vi "Requests.vi"(8 "error in (no error)":errorcluster, 9 "write enable":bool=TRUE, 11 "TCP Client in":refnum<class "WebSocket Client CR.lvclass">) -> (0 "error out":errorcluster, 3 "MB_TCP out":refnum<class "WebSocket Client CR.lvclass">)   [LabVIEW 2021, in "WebSockets.lvlib" / "WebSocket Client CR.lvclass"]
uses:
  WebSocket Client CR.lvclass
  WebSocket/WebSocket.lvclass
  WebSocket Server/TCP Server/Handler State.ctl
  WebSocket Server/TCP Server/TCP Server.lvclass
  WebSocket/Opcodes.ctl
  Data Model/WebSocket Data Model.lvclass
  Modbus_v121c/Data Model/Device Data Model.lvclass
panel:
  out "Data":u8[](array[numeric])
  in  "stop":bool
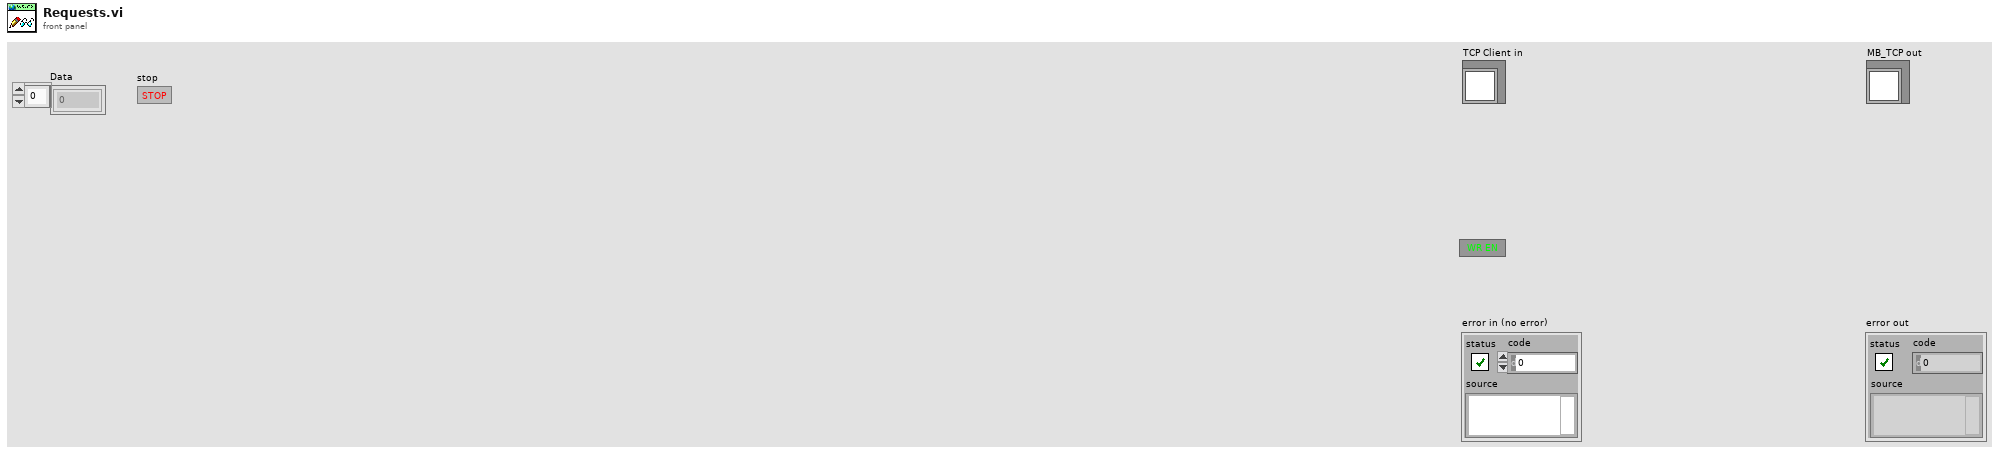
[diagram p1: front panel]
types:
  T1 = typedef "WebSockets.lvlib/WebSocket.lvclass/Opcodes.ctl" = u8
  T2 = typedef "WebSockets.lvlib/TCP Server.lvclass/Handler State.ctl" = enum16{"Wait on Connection", "Execute function", "Close Connection", "Quit"}
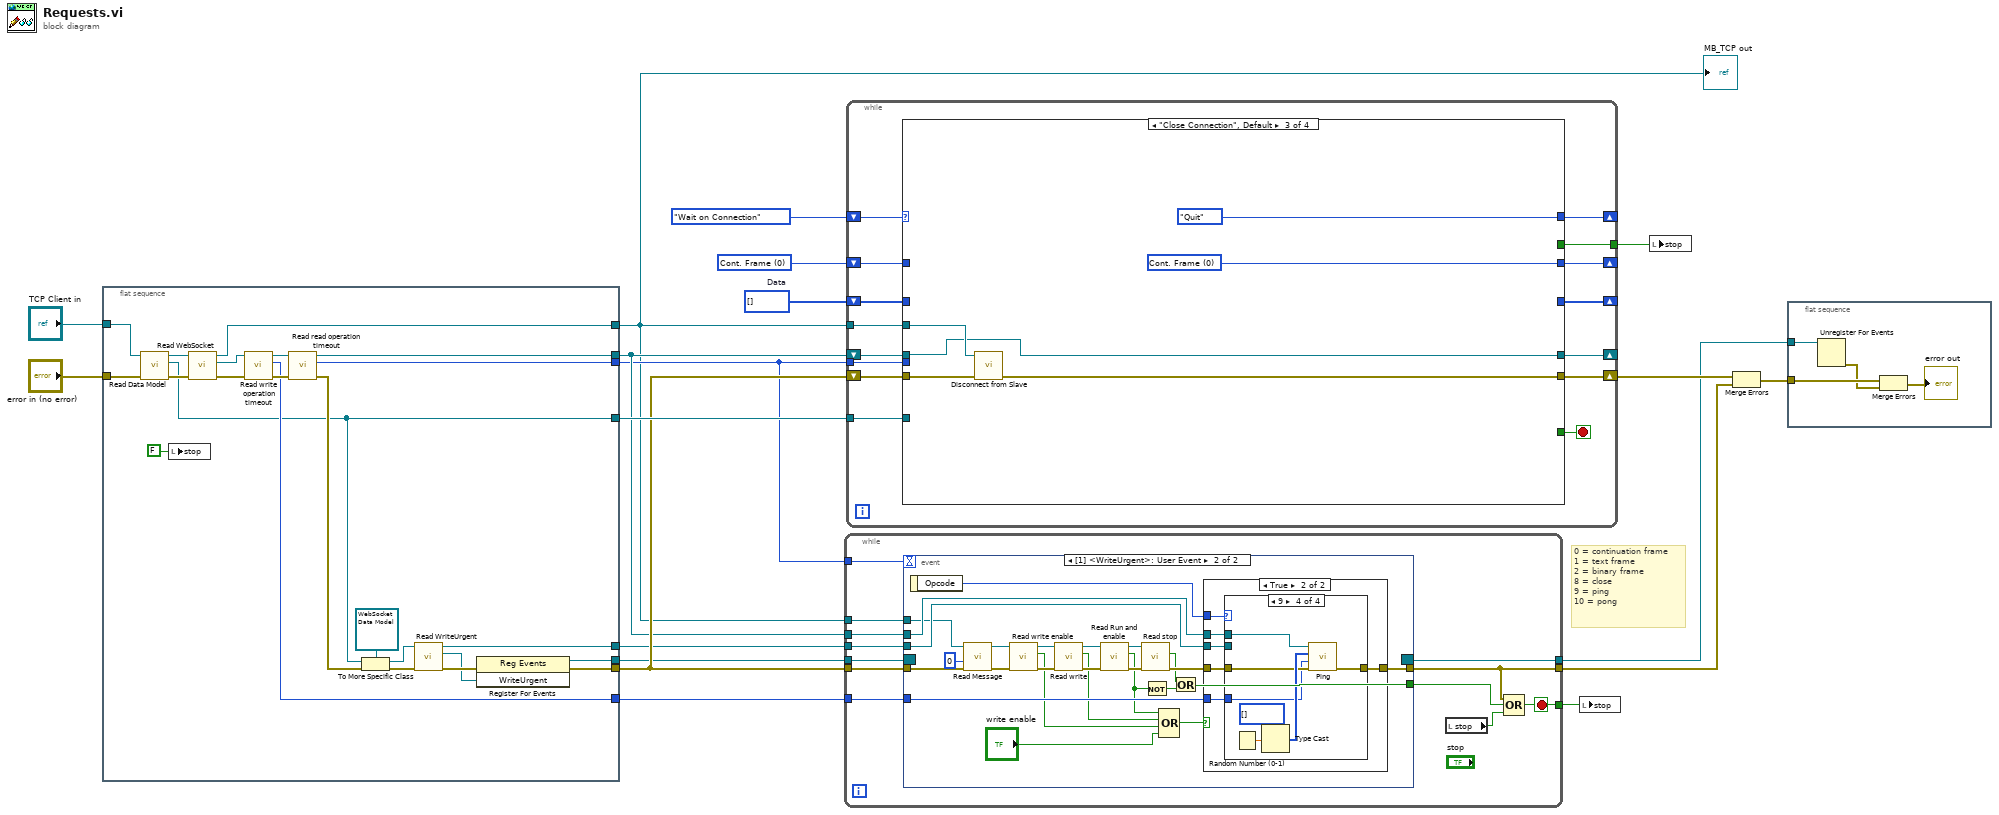
[diagram p0: block diagram]
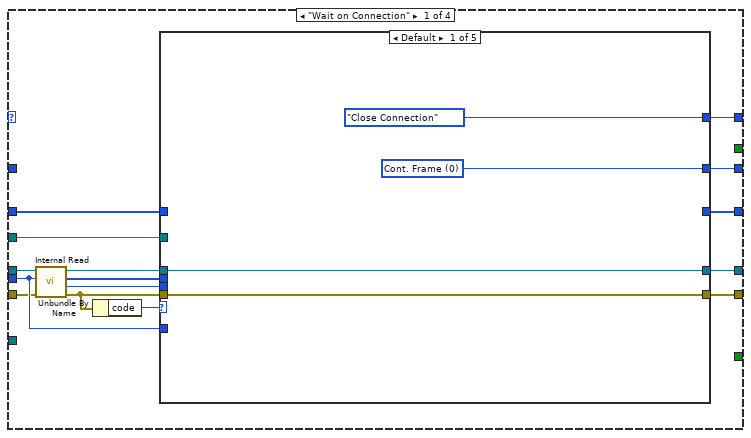
[diagram p2: hidden frame]
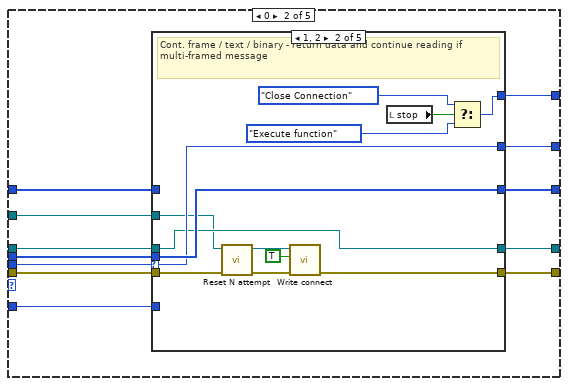
[diagram p3: hidden frame]
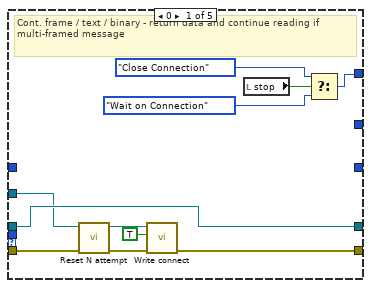
[diagram p4: hidden frame]
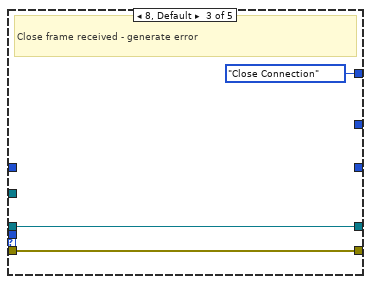
[diagram p5: hidden frame]
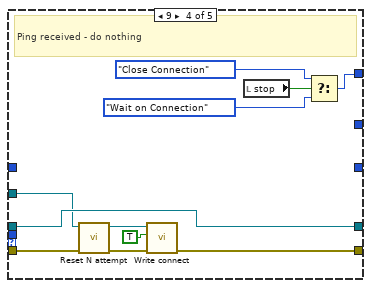
[diagram p6: hidden frame]
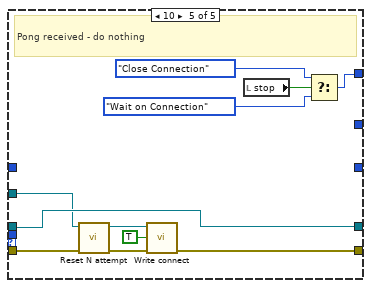
[diagram p7: hidden frame]
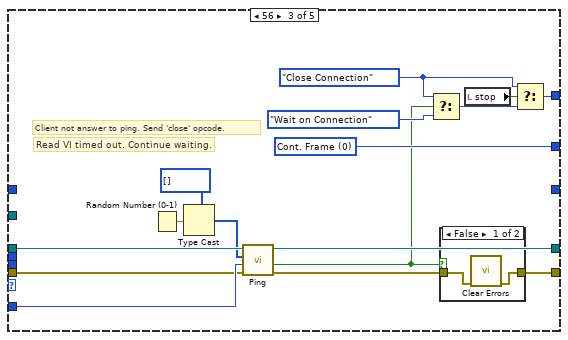
[diagram p8: hidden frame]
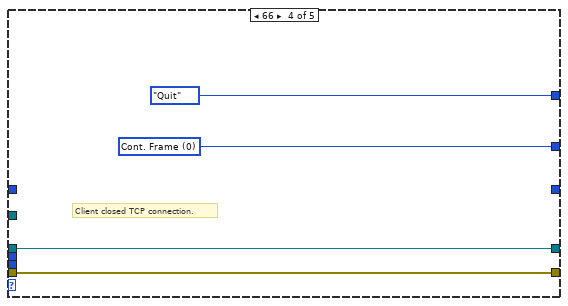
[diagram p10: hidden frame]
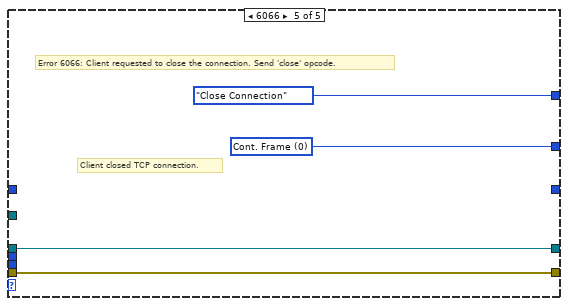
[diagram p11: hidden frame]
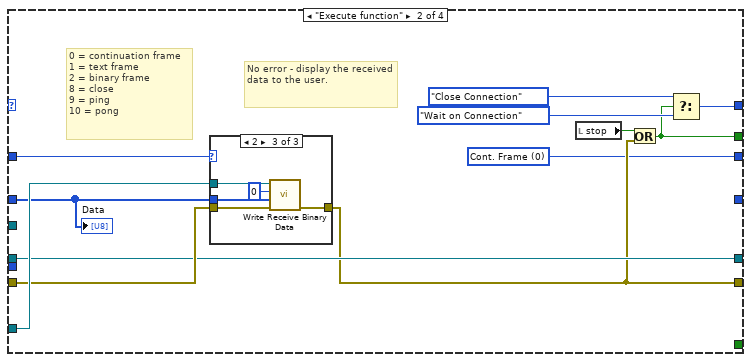
[diagram p12: hidden frame]
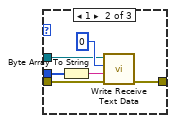
[diagram p14: hidden frame]
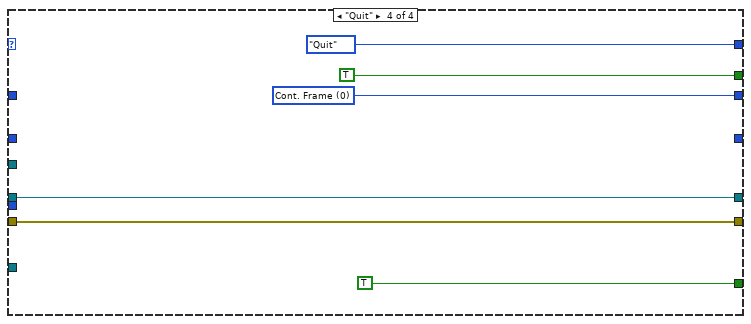
[diagram p15: hidden frame]
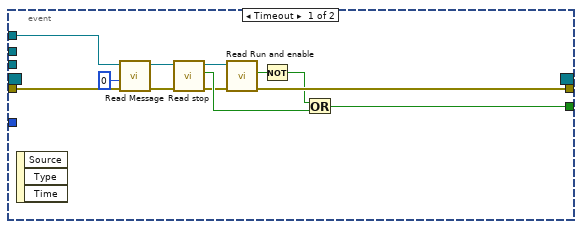
[diagram p16: hidden frame]
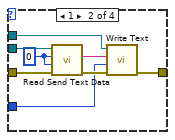
[diagram p19: hidden frame]
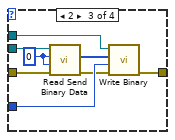
[diagram p20: hidden frame]
diagram:
  w7 = T1 0 items=["Cont. Frame"=0, "Text"=1, "Binary"=2, "Close Frame"=8, "Ping"=9, "Pong"=10] ("Opcode")
  w19 = u8[] []  # Data
  # "0 = continuation frame\n1 = text frame\n2 = binary frame\n8 = close\n9 = ping\n10 = pong"
  n1 = flat-sequence {
    tunnel: [w29] -> w14
    tunnel: [w41] -> w6
    tunnel: [w37] -> w13
    tunnel: [w20] -> w15
    tunnel: [w28] -> w8
    tunnel: [w34] -> w11
    tunnel: [w32] -> w12
    tunnel: [w21] -> w1
    tunnel: "TCP Client in" -> [w23]
    tunnel: "error in (no error)" -> [w25]
    frame #0 {
      n2 = call "Read Data Model.vi"("error in (no error)"=w25, "Master CR in"=w23) -> ("error out"=w24:errorcluster, "Data Model"=w20:refnum<class "Device Data Model.lvclass">, "Master CR out"=w22:refnum<class "WebSocket Client CR.lvclass">)  [unwired: 7 in]
      n3 = local write "stop"(FALSE ("stop")) -> ()
      n4 = call "Read WebSocket.vi"("error in (no error)"=w24, "Master CR in"=w22) -> ("error out"=w26:errorcluster, "WebSocket"=w27:refnum<class "WebSocket.lvclass">, "Master CR out"=w21:refnum<class "WebSocket Client CR.lvclass">)  [unwired: 7 in]
      n5 = call "Read write operation timeout.vi"("error in (no error)"=w26, "Socket in"=w27) -> ("error out"=w35:errorcluster, "write operation timeout"=w34:i32, "Socket out"=w36:refnum<class "WebSocket.lvclass">)  [unwired: 7 in]
      n6 = call "Read read operation timeout.vi"("error in (no error)"=w35, "Socket in"=w36) -> ("error out"=w33:errorcluster, "read operation timeout"=w41:i32, "Socket out"=w37:refnum<class "WebSocket.lvclass">)  [unwired: 7 in]
      n7 = To More Specific Class(target class=refnum<class "WebSocket Data Model.lvclass"> refnum ("WebSockets.lvlib:Device Data Model"), reference=w20, error in=w33) -> (specific class reference=w39:refnum<class "WebSocket Data Model.lvclass">, error out=w38:errorcluster)
      n8 = call "Read WriteUrgent.vi"("error in (no error)"=w38, "WebSocket Data Model in"=w39) -> ("error out"=w31:errorcluster, "WriteUrgent"=w30:refnum<user-event>, "WebSocket Data Model out"=w32:refnum<class "WebSocket Data Model.lvclass">)  [unwired: 7 in]
      n9 = register-events(error in=w31, w30) -> (reference out=w28:refnum<event-registration>, error out=w29:errorcluster)  [unwired: 1 in]
    }
  }
  n10 = while {
    tunnel: [w53] -> w10
    tunnel: [w44] -> w9
    tunnel: w8 -> [w48]
    tunnel: w14 -> [w52]
    tunnel: w13 -> [w51]
    tunnel: w12 -> [w50]
    tunnel: w11 -> [w49]
    tunnel: w1 -> [w47]
    tunnel: w6 -> [w46]
    tunnel: [w43] -> w5
    stop <- w53 stop-if-true
    n11 = event shown="[1] <WriteUrgent>: User Event" {
      selector: w48 -> [_ _]
      dyn-events: [_ _] -> w43
      timeout: w46 -> [_ _]
      tunnel: w52 -> [w63 w78]
      tunnel: w51 -> [_ w88]
      tunnel: w50 -> [_ w87]
      tunnel: [w58 w91] -> w44
      tunnel: w49 -> [_ w90]
      tunnel: w47 -> [w62 w75]
      tunnel: [w57 w67] -> w45
      event Timeout {
        n12 = event-data() -> ()  [unwired: 1 in, 3 out]
        n13 = call "Read Message.vi"("error in (no error)"=w63, "timeout (0)"=0, "Master CR in"=w62) -> ("error out"=w64:errorcluster, "Master CR out"=w61:refnum<class "WebSocket Client CR.lvclass">)  [unwired: 6 in, 1 out]
        n14 = call "Read stop.vi"("error in (no error)"=w64, "Master CR in"=w61) -> ("error out"=w60:errorcluster, "Stop"=w66:bool, "Master CR out"=w59:refnum<class "WebSocket Client CR.lvclass">)  [unwired: 7 in]
        n15 = call "Read Run and enable.vi"("error in (no error)"=w60, "Master CR in"=w59) -> ("error out"=w58:errorcluster, "Enable and Run"=w56:bool)  [unwired: 7 in, 1 out]
        n16 = Not(x=w56) -> (.not. x?=w55:bool)
        n17 = Or(x=w55, y=w66) -> (x .or. y?=w57:bool)
      }
      event User Event {
        n18 = event-data() -> ("Opcode"=w89:T1)  [unwired: 1 in]
        n19 = call "Read Message.vi"("error in (no error)"=w78, "timeout (0)"=0, "Master CR in"=w75) -> ("error out"=w77:errorcluster, "Master CR out"=w76:refnum<class "WebSocket Client CR.lvclass">)  [unwired: 6 in, 1 out]
        n20 = call "Read write enable.vi"("error in (no error)"=w77, "Master CR in"=w76) -> ("error out"=w84:errorcluster, "write enable"=w80:bool, "Master CR out"=w83:refnum<class "WebSocket Client CR.lvclass">)  [unwired: 7 in]
        n21 = call "Read write.vi"("error in (no error)"=w84, "Master CR in"=w83) -> ("error out"=w85:errorcluster, "Write"=w81:bool, "Master CR out"=w86:refnum<class "WebSocket Client CR.lvclass">)  [unwired: 7 in]
        n22 = call "Read Run and enable.vi"("error in (no error)"=w85, "Master CR in"=w86) -> ("error out"=w73:errorcluster, "Enable and Run"=w70:bool, "Master CR out"=w72:refnum<class "WebSocket Client CR.lvclass">)  [unwired: 7 in]
        n23 = call "Read stop.vi"("error in (no error)"=w73, "Master CR in"=w72) -> ("error out"=w71:errorcluster, "Stop"=w68:bool)  [unwired: 7 in, 1 out]
        n24 = Not(x=w70) -> (.not. x?=w69:bool)
        n25 = Compound Arithmetic op=OR(w70, w81, w80, "write enable") -> (w82:bool)
        n26 = Or(x=w68, y=w69) -> (x .or. y?=w67:bool)
        n27 = case shown="True" w82 {
          tunnel: w88 -> [_ w98]
          tunnel: w87 -> [_ w97]
          tunnel: [w92 w96] -> w91
          tunnel: w90 -> [_ w95]
          tunnel: w71 -> [w92 w94]
          tunnel: w89 -> [_ w93]
          frame False {
          }
          frame True {
            n28 = case shown="9" w93 {
              tunnel: w98 -> [_ w107 w115 w120]
              tunnel: w94 -> [w99 w106 w111 w118]
              tunnel: w97 -> [_ w105 w112 _]
              tunnel: w95 -> [_ w101 w113 w116]
              tunnel: [w99 w100 w114 w117] -> w96
              frame 0, Default {
              }
              frame 1 {
                w104 = u16 0 ("starting address")
                n29 = call-dynamic "Read Send Text Data.vi"("error in (no error)"=w106, "number of registers"=w104, "starting address"=w104, "device data model in"=w105) -> ("error out"=w102:errorcluster, "data"=w103:string)  [unwired: 5 in, 1 out]
                n30 = call-dynamic "Write Text.vi"("error in (no error)"=w102, "timeout ms (5000)"=w101, "String Data"=w103, "WebSocket in"=w107) -> ("error out"=w100:errorcluster)  [unwired: 6 in, 1 out]
              }
              frame 2 {
                w108 = u16 0 ("starting address")
                n31 = call-dynamic "Read Send Binary Data.vi"("error in (no error)"=w111, "number of registers"=w108, "starting address"=w108, "device data model in"=w112) -> ("error out"=w109:errorcluster, "data"=w110:u8[])  [unwired: 5 in, 1 out]
                n32 = call-dynamic "Write Binary.vi"("error in (no error)"=w109, "timeout ms (5000)"=w113, "Binary Data"=w110, "WebSocket in"=w115) -> ("error out"=w114:errorcluster)  [unwired: 6 in, 1 out]
              }
              frame 9 {
                n33 = Random Number (0-1)() -> (number: 0 to 1=w121:dbl)
                n34 = Type Cast(type=u8[] [] ("values"), x=w121) -> (*(type *) &x=w119:u8[])
                n35 = call "Ping.vi"("error in (no error)"=w118, "timeout ms (5000)"=w116, "Payload"=w119, "WebSocket in"=w120) -> ("error out"=w117:errorcluster)  [unwired: 5 in, 2 out]
              }
            }
          }
        }
      }
    }
    n36 = local read "stop"() -> (w54:bool)
    n37 = Compound Arithmetic op=OR(w44, w45, w54) -> (w53:bool)
  }
  n38 = while {
    tunnel: w6 -> [w135]
    shift-right: [w136] -> _
    shift-left: w13 -> [w137]
    shift-right: [w133] -> _
    shift-left: w19 -> [w134]
    shift-right: [w123] -> _
    shift-left: Handler_State."Wait on Connection" ("Listener State") -> [w132]
    tunnel: [w124] -> w17
    shift-right: [w129] -> w16
    shift-left: w14 -> [w131]
    tunnel: w15 -> [w128]
    shift-right: [w127] -> _
    shift-left: w7 -> [w126]
    tunnel: w1 -> [w125]
    stop <- w130 stop-if-true
    n39 = case shown="\"Close Connection\", Default" w132 {
      tunnel: w137 -> [w147 w253 w270 w279]
      tunnel: [w152 w252 w269 w277] -> w129
      tunnel: [w151 w253 w270 w279] -> w136
      tunnel: [_ _ _ TRUE ("Finished?")] -> w130
      tunnel: w135 -> [w144 _ _ _]
      tunnel: w134 -> [w150 w255 _ _]
      tunnel: [w149 _ _ _] -> w133
      tunnel: w131 -> [w143 w254 w272 w277]
      tunnel: w128 -> [_ w256 _ _]
      tunnel: [w140 w251 w274 w278] -> w127
      tunnel: w126 -> [_ w250 _ _]
      tunnel: w125 -> [w139 _ w271 _]
      tunnel: [_ w246 _ TRUE] -> w124
      tunnel: [w138 w245 Handler_State."Quit" ("Listener State") Handler_State."Quit" ("Listener State")] -> w123
      frame "Wait on Connection" {
        n40 = call "Internal Read.vi"("error in (no error)"=w143, "timeout ms"=w144, "WebSocket in"=w147) -> ("error out"=w142:errorcluster, "Opcode"=w141:T1, "Data"=w145:u8[], "WebSocket out"=w146:refnum<class "WebSocket.lvclass">)  [unwired: 5 in]
        n41 = Unbundle By Name(w142) -> ("code"=w148:i32)
        n42 = case shown="Default" w148 {
          tunnel: w142 -> [w156 w168 w223 w237 w241]
          tunnel: [w156 w167 w233 w237 w241] -> w152
          tunnel: w146 -> [w155 w166 w232 w240 w244]
          tunnel: w145 -> [_ w165 _ _ _]
          tunnel: [w155 w164 w224 w240 w244] -> w151
          tunnel: w141 -> [_ w163 _ _ _]
          tunnel: w144 -> [_ w162 w231 _ _]
          tunnel: w150 -> [_ w161 _ _ _]
          tunnel: [_ w160 _ _ _] -> w149
          tunnel: [Handler_State."Close Connection" ("Listener State") w159 w218 Handler_State."Quit" ("Listener State") Handler_State."Close Connection" ("Listener State")] -> w138
          tunnel: [w153 w158 w229 w238 w242] -> w140
          tunnel: w139 -> [_ w157 _ _ _]
          frame Default {
            w153 = T1 0 items=["Cont. Frame", "Text", "Binary", "Close Frame", "Ping", "Pong"] ("Opcode")
          }
          frame 0 {
            n43 = case shown="1, 2" w163 {
              selector: w163 -> [_ w191 _ _ _]
              tunnel: w168 -> [w174 w185 w195 w203 w214]
              tunnel: [w173 w184 w195 w201 w213] -> w167
              tunnel: w166 -> [w176 w187 w194 w202 w212]
              tunnel: w165 -> [_ w192 _ _ _]
              tunnel: [w176 w187 w194 w202 w212] -> w164
              tunnel: w162 -> [_ _ _ _ _]
              tunnel: w161 -> [_ _ _ _ _]
              tunnel: [_ w192 _ _ _] -> w160
              tunnel: [w169 w180 Handler_State."Close Connection" ("Listener State") w196 w207] -> w159
              tunnel: [_ w191 _ _ _] -> w158
              tunnel: w157 -> [w175 w186 _ w200 w211]
              frame 0 {
                # "Cont. frame / text / binary - return data and continue reading if multi-framed message"
                n44 = call "Reset N attempt.vi"("error in (no error)"=w174, "Master CR in"=w175) -> ("error out"=w178:errorcluster, "Master CR out"=w179:refnum<class "WebSocket Client CR.lvclass">)  [unwired: 8 in]
                n45 = call "Write connect.vi"("error in (no error)"=w178, "connect"=TRUE, "Master CR in"=w179) -> ("error out"=w173:errorcluster)  [unwired: 7 in, 1 out]
                n46 = local read "stop"() -> (w172:bool)
                n47 = Select(t=Handler_State."Close Connection" ("Listener State"), s=w172, f=Handler_State."Wait on Connection" ("Listener State")) -> (s? t:f=w169:T2)
              }
              frame 1, 2 {
                # "Cont. frame / text / binary - return data and continue reading if multi-framed message"
                n48 = call "Reset N attempt.vi"("error in (no error)"=w185, "Master CR in"=w186) -> ("error out"=w189:errorcluster, "Master CR out"=w190:refnum<class "WebSocket Client CR.lvclass">)  [unwired: 8 in]
                n49 = call "Write connect.vi"("error in (no error)"=w189, "connect"=TRUE, "Master CR in"=w190) -> ("error out"=w184:errorcluster)  [unwired: 7 in, 1 out]
                n50 = local read "stop"() -> (w183:bool)
                n51 = Select(t=Handler_State."Close Connection" ("Listener State"), s=w183, f=Handler_State."Execute function" ("Listener State")) -> (s? t:f=w180:T2)
              }
              frame 8, Default {
                # "Close frame received - generate error"
              }
              frame 9 {
                # "Ping received - do nothing"
                n52 = call "Reset N attempt.vi"("error in (no error)"=w203, "Master CR in"=w200) -> ("error out"=w205:errorcluster, "Master CR out"=w206:refnum<class "WebSocket Client CR.lvclass">)  [unwired: 8 in]
                n53 = call "Write connect.vi"("error in (no error)"=w205, "connect"=TRUE, "Master CR in"=w206) -> ("error out"=w201:errorcluster)  [unwired: 7 in, 1 out]
                n54 = local read "stop"() -> (w199:bool)
                n55 = Select(t=Handler_State."Close Connection" ("Listener State"), s=w199, f=Handler_State."Wait on Connection" ("Listener State")) -> (s? t:f=w196:T2)
              }
              frame 10 {
                # "Pong received - do nothing"
                n56 = call "Reset N attempt.vi"("error in (no error)"=w214, "Master CR in"=w211) -> ("error out"=w216:errorcluster, "Master CR out"=w217:refnum<class "WebSocket Client CR.lvclass">)  [unwired: 8 in]
                n57 = call "Write connect.vi"("error in (no error)"=w216, "connect"=TRUE, "Master CR in"=w217) -> ("error out"=w213:errorcluster)  [unwired: 7 in, 1 out]
                n58 = local read "stop"() -> (w210:bool)
                n59 = Select(t=Handler_State."Close Connection" ("Listener State"), s=w210, f=Handler_State."Wait on Connection" ("Listener State")) -> (s? t:f=w207:T2)
              }
            }
          }
          frame 56 {
            w219 = Handler_State."Close Connection" ("Listener State")
            w229 = T1 0 items=["Cont. Frame", "Text", "Binary", "Close Frame", "Ping", "Pong"] ("Opcode")
            # "Client not answer to ping. Send 'close' opcode."
            # "Read VI timed out. Continue waiting."
            n60 = Random Number (0-1)() -> (number: 0 to 1=w227:dbl)
            n61 = Type Cast(type=u8[] [] ("values"), x=w227) -> (*(type *) &x=w226:u8[])
            n62 = call "Ping.vi"("error in (no error)"=w223, "timeout ms (5000)"=w231, "Payload"=w226, "WebSocket in"=w232) -> ("error out"=w225:errorcluster, "timed out?"=w222:bool, "WebSocket out"=w224:refnum<class "WebSocket.lvclass">)  [unwired: 5 in]
            n63 = Select(t=w219, s=w222, f=Handler_State."Wait on Connection" ("Listener State")) -> (s? t:f=w220:T2)
            n64 = case shown="False" w222 {
              tunnel: [w235 w236] -> w233
              tunnel: w225 -> [w234 w236]
              frame False {
                n65 = call <vilib>:"Clear Errors.vi"("error in (no error)"=w234) -> ("error out"=w235:errorcluster)  [unwired: 5 in, 1 out]
              }
              frame True {
              }
            }
            n66 = local read "stop"() -> (w221:bool)
            n67 = Select(t=w219, s=w221, f=w220) -> (s? t:f=w218:T2)
          }
          frame 66 {
            w238 = T1 0 items=["Cont. Frame", "Text", "Binary", "Close Frame", "Ping", "Pong"] ("Opcode")
            # "Client closed TCP connection."
          }
          frame 6066 {
            w242 = T1 0 items=["Cont. Frame", "Text", "Binary", "Close Frame", "Ping", "Pong"] ("Opcode")
            # "Error 6066: Client requested to close the connection. Send 'close' opcode."
            # "Client closed TCP connection."
          }
        }
      }
      frame "Execute function" {
        w251 = T1 0 items=["Cont. Frame", "Text", "Binary", "Close Frame", "Ping", "Pong"] ("Opcode")
        # "0 = continuation frame\n1 = text frame\n2 = binary frame\n8 = close\n9 = ping\n10 = pong"
        # "No error - display the received data to the user."
        n68 = case shown="2" w250 {
          tunnel: w255 -> [_ w263 w265]
          tunnel: w256 -> [_ w259 w266]
          tunnel: w254 -> [w257 w262 w268]
          tunnel: [w257 w258 w267] -> w252
          frame 0, Default {
          }
          frame 1 {
            n69 = Byte Array To String(unsigned byte array=w263) -> (string=w260:string)
            n70 = call-dynamic "Write Receive Text Data.vi"("error in (no error)"=w262, "values"=w260, "starting address"=u16 0, "standard data model in"=w259) -> ("error out"=w258:errorcluster)  [unwired: 6 in, 1 out]
          }
          frame 2 {
            n71 = call-dynamic "Write Receive Binary Data.vi"("error in (no error)"=w268, "values"=w265, "starting address"=u16 0, "standard data model in"=w266) -> ("error out"=w267:errorcluster)  [unwired: 6 in, 1 out]
          }
        }
        n72 = local read "stop"() -> (w249:bool)
        n73 = Or(x=w249, y=w252) -> (x .or. y?=w246:bool)
        n74 = Select(t=Handler_State."Close Connection" ("Listener State"), s=w246, f=Handler_State."Wait on Connection" ("Listener State")) -> (s? t:f=w245:T2)
        "Data" <- w255
      }
      frame "Close Connection", Default {
        w274 = T1 0 items=["Cont. Frame", "Text", "Binary", "Close Frame", "Ping", "Pong"] ("Opcode")
        n75 = call-dynamic "Disconnect from Slave.vi"("error in (no error)"=w272, "network master in"=w271) -> ("error out"=w269:errorcluster)  [unwired: 8 in, 1 out]
      }
      frame "Quit" {
        w278 = T1 0 items=["Cont. Frame", "Text", "Binary", "Close Frame", "Ping", "Pong"] ("Opcode")
      }
    }
  }
  n76 = local write "stop"(w10) -> ()
  n77 = local write "stop"(w17) -> ()
  n78 = Merge Errors(w16, w9) -> (w4:errorcluster)
  n79 = flat-sequence {
    tunnel: w5 -> [w282]
    tunnel: w4 -> [w284]
    frame #0 {
      n80 = Unregister For Events(event registration refnum=w282) -> (error out=w283:errorcluster)  [unwired: 1 in]
      n81 = Merge Errors(w284, w283) -> (→"error out":errorcluster)
    }
  }
  "MB_TCP out" <- w1
